vi "Main_GOOP3_ActiveObject_Debugger_Open_GDS.vi"() -> ()   [LabVIEW 2016]
doc: "This Main VI show how to create Active objects and use the debugger"
uses:
  Map_class/Map.lvclass
  Object_class/Object.lvclass
  Object_class/protected/Walkabout.vi
panel:
  in  "Objects To Create":i32=5
  in  "Stop":bool
  out "error out":errorcluster
  out "Mace":picture
  # "Objects in a maze"
  # "Start the application to show X number of creatures\nrun around in the maze.\n\nEvery creature is running a background process.\nThis process is controlling the induvidual creatures\nmovements in the maze."
  # "To debug the objects open the debugger dialog\nTools->GOOP->Debuggers->Object Debugger\n\n-View the data of an object\n-Try to update the color of an existing object.\n\nView more information here:\nhttp://goop.endevo.net/GDS/videos/Debugger/"
  # "Every object runs a\n\"Walkabout\" process\nthat changes the \nposition of the \"Object\""
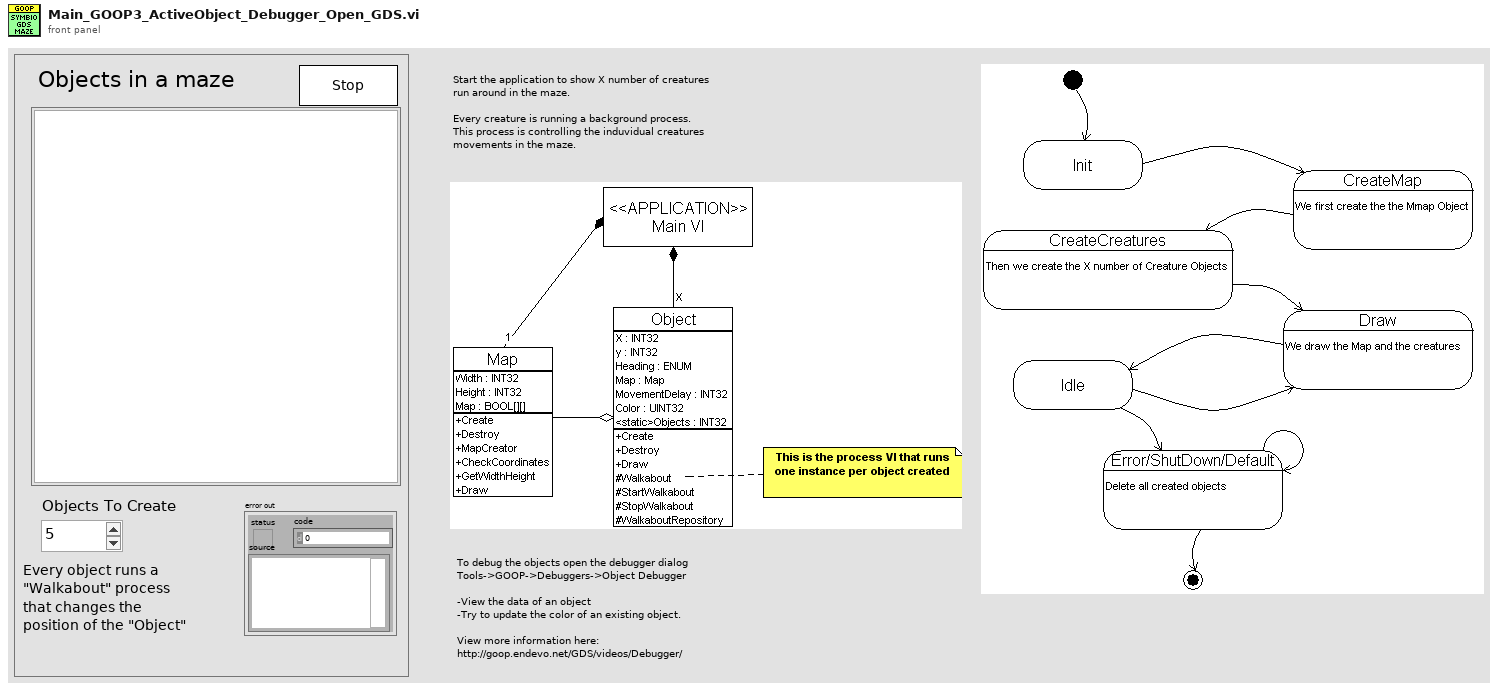
[diagram p1: front panel]
types:
  T1 = cluster{"Map":refnum<class "Map.lvclass">, "Objects":refnum<class "Object.lvclass">[]}
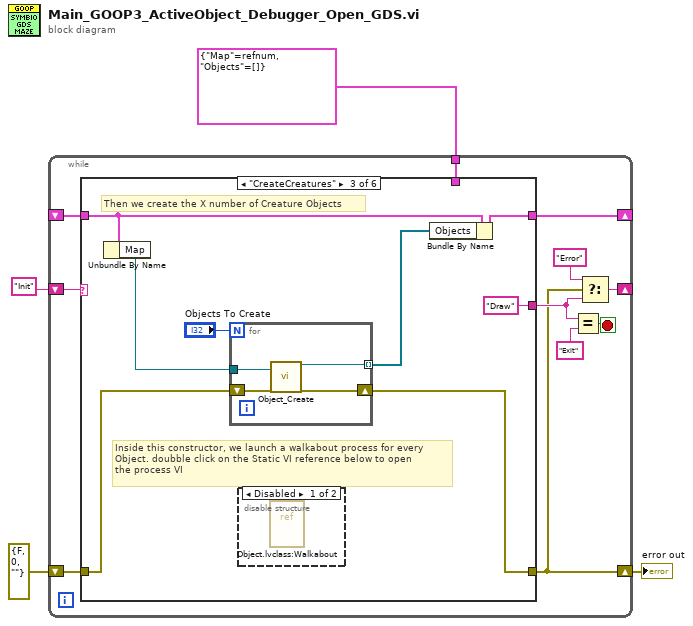
[diagram p0: block diagram]
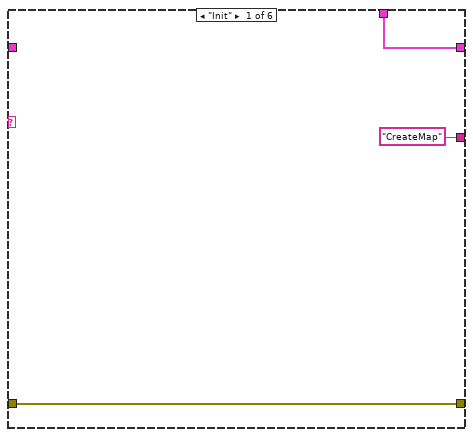
[diagram p2: hidden frame]
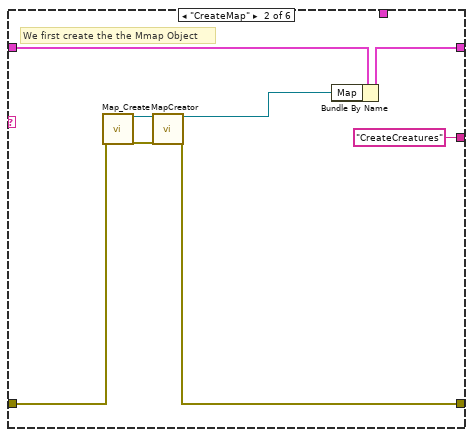
[diagram p3: hidden frame]
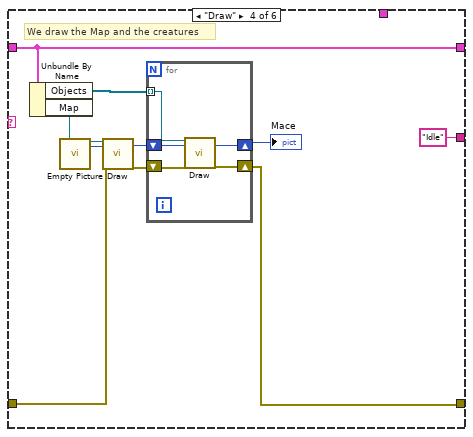
[diagram p5: hidden frame]
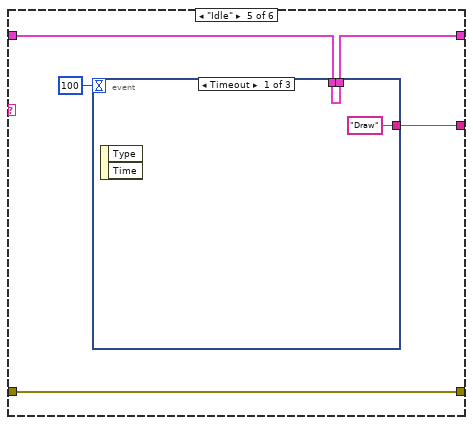
[diagram p6: hidden frame]
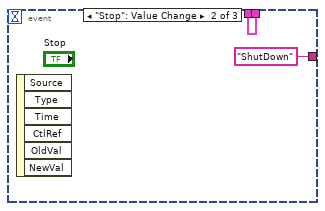
[diagram p7: hidden frame]
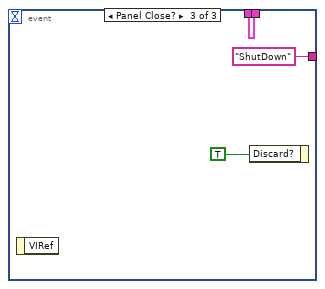
[diagram p8: hidden frame]
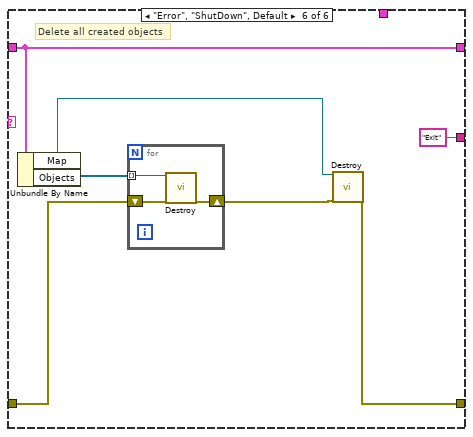
[diagram p9: hidden frame]
diagram:
  n1 = while {
    shift-right: [w8] -> w2
    shift-left: errorcluster {"status"=FALSE, "code"=0, "source"=""} ("error IO") -> [w15]
    shift-right: [w13] -> _
    shift-left: "Init" -> [w14]
    shift-right: [w7] -> _
    shift-left: _ -> [w6]
    tunnel: T1 {"Map"=refnum, "Objects"=[]} -> [w5]
    stop <- w12 stop-if-true
    n2 = case shown="\"CreateCreatures\"" w14 {
      tunnel: w15 -> [w17 w21 w33 w47 w55 w70]
      tunnel: [w17 w20 w32 w43 w55 w69] -> w8
      tunnel: ["CreateMap" "CreateCreatures" "Draw" "Idle" w56 "Exit"] -> w9
      tunnel: [w16 w24 w30 w41 w57 w66] -> w7
      tunnel: w6 -> [_ w25 w28 w41 w58 w66]
      tunnel: w5 -> [w16 _ _ _ _ _]
      frame "Init" {
      }
      frame "CreateMap" {
        # "We first create the the Mmap Object"
        n3 = call "Map_Create.vi"("error in (no error)"=w21) -> ("reference out"=w23:refnum<class "Map.lvclass">, "error out"=w22:errorcluster)  [unwired: 17 out]
        n4 = call-dynamic "MapCreator.vi"("reference in"=w23, "error in (no error)"=w22) -> ("reference out"=w19:refnum<class "Map.lvclass">, "error out"=w20:errorcluster)  [unwired: 1 in, 15 out]
        n5 = Bundle By Name(cluster=w25, "Map"=w19) -> (w24:T1)
      }
      frame "CreateCreatures" {
        # "Inside this constructor, we launch a walkabout process for every\nObject. doubble click on the Static VI reference below to open\nthe process VI"
        # "Then we create the X number of Creature Objects"
        n6 = Unbundle By Name(w28) -> ("Map"=w27:refnum<class "Map.lvclass">)
        n7 = for {
          N: "Objects To Create" -> [_]
          shift-right: [w37] -> w32
          shift-left: w33 -> [w38]
          tunnel: [w36] -> w31 mode=indexing
          tunnel: w27 -> [w35]
          n8 = call "Object_Create.vi"("MapRef"=w35, "error in (no error)"=w38) -> ("reference out"=w36:refnum<class "Object.lvclass">, "error out"=w37:errorcluster)  [unwired: 16 out]
        }
        n9 = disable-structure shown="Disabled" {
          frame Disabled {
            n10 = vi-ref "Object.lvclass:Walkabout.vi"() -> ()  [unwired: 1 out]
          }
          frame Enabled {
          }
        }
        n11 = Bundle By Name(cluster=w28, "Objects"=w31) -> (w30:T1)
      }
      frame "Draw" {
        # "We draw the Map and the creatures"
        n12 = Unbundle By Name(w41) -> ("Objects"=w45:refnum<class "Object.lvclass">[], "Map"=w48:refnum<class "Map.lvclass">)
        n13 = call "Empty Picture"() -> ("empty picture"=w40:picture)
        n14 = call-dynamic "Draw.vi"("reference in"=w48, "PictureIn"=w40, "error in (no error)"=w47) -> ("PictureOut"=w39:picture, "error out"=w46:errorcluster)  [unwired: 15 out]
        n15 = for {
          tunnel: w45 -> [w52] mode=indexing
          shift-right: [w50] -> w44
          shift-left: w39 -> [w51]
          shift-right: [w49] -> w43
          shift-left: w46 -> [w53]
          n16 = call-dynamic "Draw.vi"("reference in"=w52, "PictureIn"=w51, "error in (no error)"=w53) -> ("PictureOut"=w50:picture, "error out"=w49:errorcluster)  [unwired: 15 out]
        }
        "Mace" <- w44
      }
      frame "Idle" {
        n17 = event shown="[0] Timeout" {
          selector: _ -> [_ _ _]
          dyn-events: _ -> [_ _ _]
          timeout: 100 -> [_ _ _]
          tunnel: w58 -> [w59 w61 w63]
          tunnel: [w59 w61 w63] -> w57
          tunnel: ["Draw" "ShutDown" "ShutDown"] -> w56
          event Timeout {
            n18 = event-data() -> ()  [unwired: 3 out]
          }
          event "Stop": Value Change {
            n19 = event-data() -> ()  [unwired: 7 out]
          }
          event Panel Close? {
            n20 = event-data() -> ()  [unwired: 2 out]
            n21 = event-data("Discard?"=TRUE) -> ()  [unwired: 1 in, 1 out]
          }
        }
      }
      frame "Error", "ShutDown", Default {
        # "Delete all created objects"
        n22 = Unbundle By Name(w66) -> ("Map"=w68:refnum<class "Map.lvclass">, "Objects"=w72:refnum<class "Object.lvclass">[])
        n23 = for {
          tunnel: w72 -> [w75] mode=indexing
          shift-right: [w74] -> w71
          shift-left: w70 -> [w73]
          n24 = call-dynamic "Destroy.vi"("reference in"=w75, "error in (no error)"=w73) -> ("error out"=w74:errorcluster)  [unwired: 17 out]
        }
        n25 = call-dynamic "Destroy.vi"("reference in"=w68, "error in (no error)"=w71) -> ("error out"=w69:errorcluster)  [unwired: 17 out]
      }
    }
    n26 = Equal?(x=w9, y="Exit") -> (x = y?=w12:bool)
    n27 = Select(t="Error", s=w8, f=w9) -> (s? t:f=w13:string)
  }
  "error out" <- w2
